vi "Shift  Master_OLD.vi"(8 "error in (no error)":errorcluster) -> (0 "error out":errorcluster)   [LabVIEW 2017]
uses:
  <vilib>/Utility/miscctls.llb/LVRowAndColumnTypeDef.ctl
  <vilib>/Utility/miscctls.llb/LVBoundsTypeDef.ctl
  <vilib>/addons/database/Connection.llb/DB Tools Open Connec (Path).vi
  Globle/Current date.vi
  <vilib>/addons/database/NI_Database_API.lvlib
panel:
  in  "Back 2":bool
  in  "UPDATE":bool
  in  "Shift 3 Stop Time":timestamp format="%<%H-%M-%S>T"
  in  "Shift 2Stop Time":timestamp format="%<%H-%M-%S>T"
  out "Shift 3 Start Time":timestamp format="%<%H-%M-%S>T"
  out "Shift 2 Start Time":timestamp format="%<%H-%M-%S>T"
  in  "Shift 1 Stop Time":timestamp format="%<%H-%M-%S>T"
  in  "Shift 1 Start time":timestamp format="%<%H-%M-%S>T"
  # "Shift Master"
  # "Shift Start Time"
  # "Shift End Time"
  # "Update"
  # "Shift Name"
  # "Shift One"
  # "Shift Two"
  # "Shift Three"
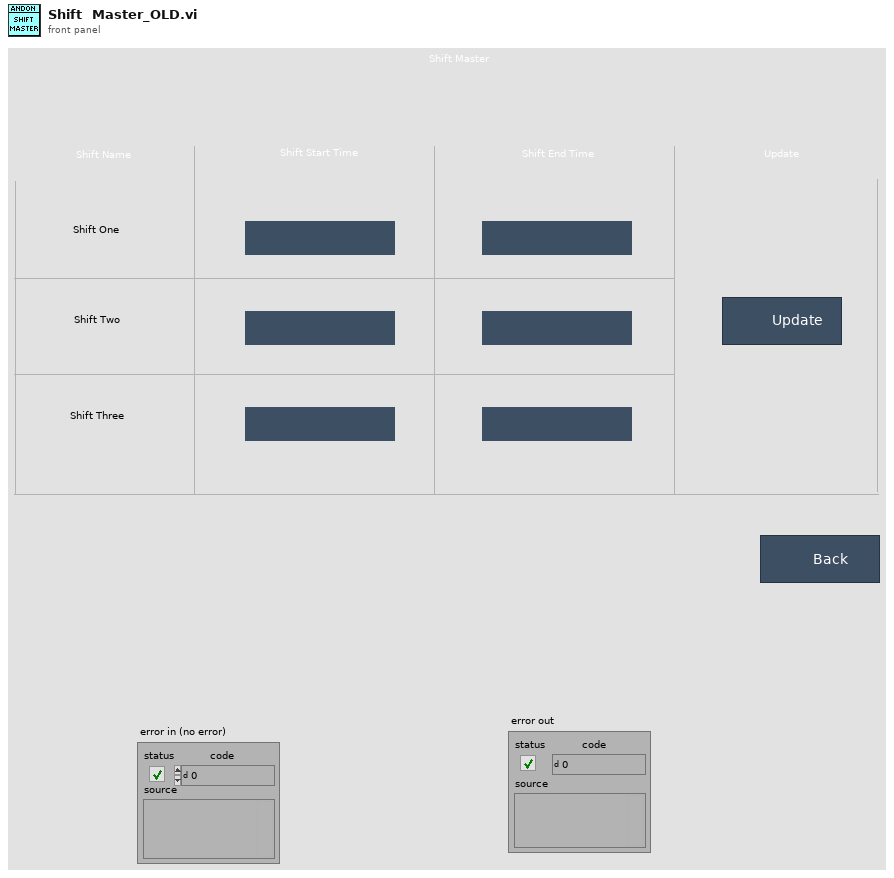
[diagram p1: front panel]
types:
  T1 = typedef "LVBoundsTypeDef.ctl" = cluster{"Width":u32, "Height":u32}
  T2 = typedef "LVRowAndColumnTypeDef.ctl" = cluster{"Row":i32, "Column":i32}
  T3 = typedef "NI_Database_API.lvlib/Conn ObjectReference.ctl" = refnum<k1>
  T4 = cluster{"Shift 3 Start Time":timestamp, "Shift 3 Stop Time ":timestamp}
  T5 = cluster{"Shift 2 Start Time":timestamp, "Shift 2Stop Time":timestamp}
  T6 = cluster{"Shift 1 Start time":timestamp, "Shift 1 Stop Time":timestamp}
  T7 = cluster{"Shift 3 Start Time":timestamp, "Shift 3 Stop Time ":timestamp}[]
  T8 = enum32{"invalid app kind", "Development System", "Run Time System", "Student Edition", "Embedded LabVIEW", "Evaluation", "Custom"}
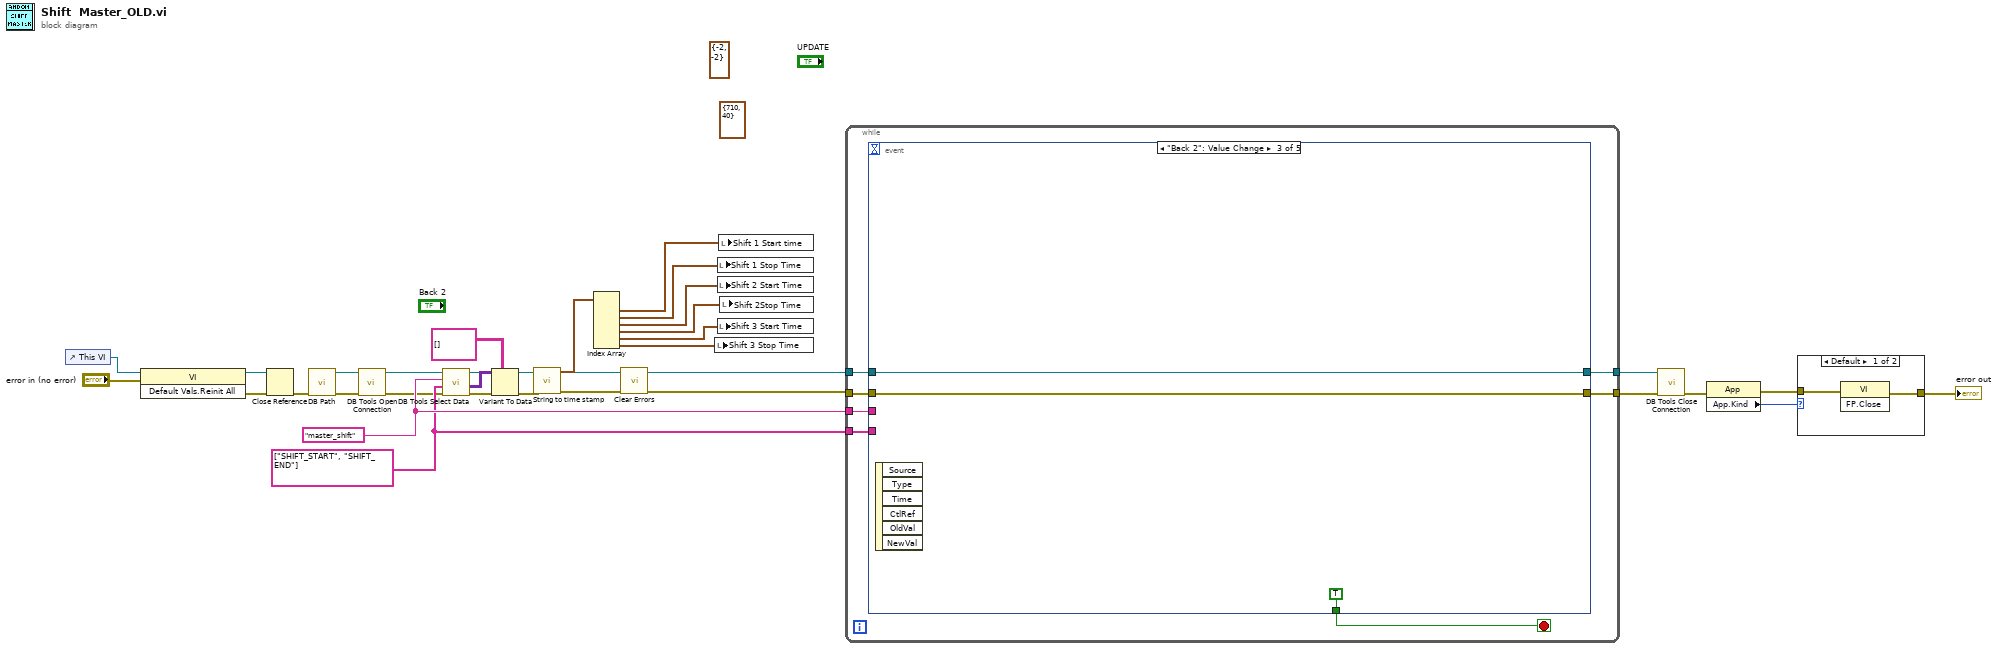
[diagram p0: block diagram]
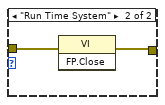
[diagram p2: hidden frame]
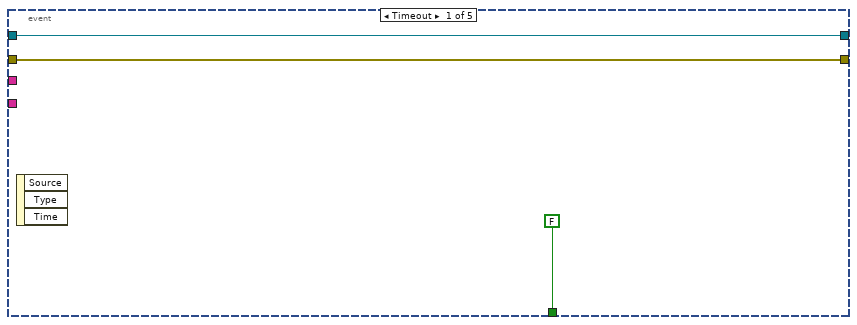
[diagram p3: hidden frame]
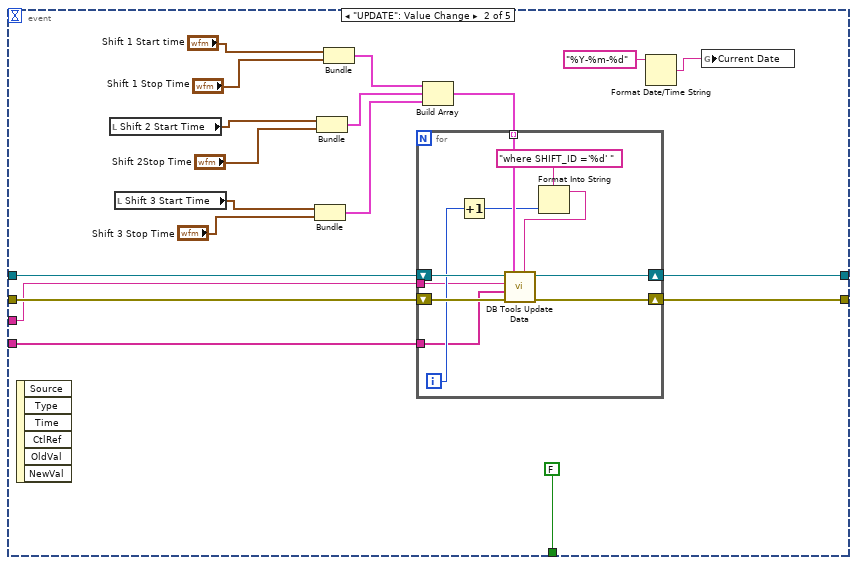
[diagram p4: hidden frame]
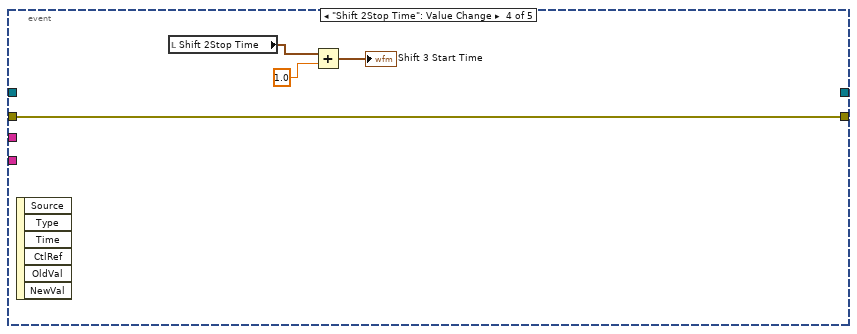
[diagram p5: hidden frame]
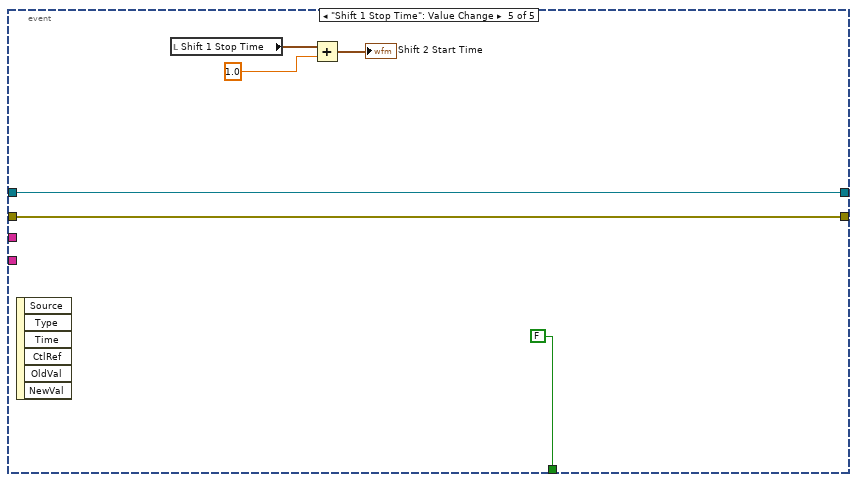
[diagram p6: hidden frame]
diagram:
  w6 = string[] ["SHIFT_START", "SHIFT_END"] ("columns")
  w7 = "master_shift" ("table")
  (unwired) T1 {"Width"=710, "Height"=40} ("Active Cell:Cell Size")
  (unwired) T2 {"Row"=-2, "Column"=-2} ("Active Cell:Active Cell")
  n1 = control-ref of="This VI"() -> (w32:refnum<vi>)
  n2 = invoke class="VI" method="Default Vals.Reinit All"(reference=w32, error in="error in (no error)") -> (reference out=w29:refnum<vi>, error out=w30:errorcluster)  [unwired: 1 in, 1 out]
  n3 = Close Reference(reference=w29, error in (no error)=w30) -> (error out=w25:errorcluster)
  n4 = call "DB Path.vi"("error in"=w25) -> ("error out"=w24:errorcluster, "DB Path"=w23:path)  [unwired: 9 in]
  n5 = call-poly <vilib>:"DB Tools Open Connection.vi"("error in (no error)"=w24, "connection information"=w23) -> ("error out"=w1:errorcluster, "connection reference"=w2:T3)  [unwired: 6 in]
  n6 = call <vilib>:"DB Tools Select Data.vi"("error in (no error)"=w1, "columns"=w6, "table"=w7, "connection reference"=w2) -> ("error out"=w21:errorcluster, "data"=w22:variant[][], "connection reference out"=w11:T3)  [unwired: 2 in]
  n7 = Variant To Data(error in=w21, type=string[][] [], Variant=w22) -> (data=w5:string[][], error out=w19:errorcluster)
  n8 = call "String to time stamp.vi"("error in (no error)"=w19, "Data In"=w5) -> ("error out"=w4:errorcluster, "Time Stamp Out"=w18:timestamp[])  [unwired: 8 in]
  n9 = Index Array(array=w18) -> (element #1=w17:timestamp, element #2=w16:timestamp, element #3=w15:timestamp, element #4=w14:timestamp, element #5=w13:timestamp, element #6=w12:timestamp)  [unwired: 6 in]
  n10 = call <vilib>:"Clear Errors.vi"("error in (no error)"=w4) -> ("error out"=w3:errorcluster)  [unwired: 5 in, 1 out]
  n11 = local write "Shift 3 Stop Time"(w12) -> ()
  n12 = local write "Shift 1 Stop Time"(w16) -> ()
  n13 = local write "Shift 2 Start Time"(w15) -> ()
  n14 = local write "Shift 3 Start Time"(w13) -> ()
  n15 = local write "Shift 1 Start time"(w17) -> ()
  n16 = local write "Shift 2Stop Time"(w14) -> ()
  n17 = while {
    tunnel: w3 -> [w39]
    tunnel: [w37] -> w10
    tunnel: w11 -> [w36]
    tunnel: [w35] -> w8
    tunnel: w7 -> [w34]
    tunnel: w6 -> [w33]
    stop <- w38 stop-if-true
    n18 = event shown="[2] \"Back 2\": Value Change" {
      selector: _ -> [_ _ _ _ _]
      dyn-events: _ -> [_ _ _ _ _]
      timeout: _ -> [_ _ _ _ _]
      tunnel: w39 -> [w41 w52 w74 w79 w83]
      tunnel: [FALSE FALSE TRUE _ FALSE] -> w38
      tunnel: [w41 w46 w74 w79 w83] -> w37
      tunnel: w36 -> [w42 w51 w75 _ w80]
      tunnel: [w42 w45 w75 _ w80] -> w35
      tunnel: w34 -> [_ w50 _ _ _]
      tunnel: w33 -> [_ w49 _ _ _]
      event Timeout {
        n19 = event-data() -> ()  [unwired: 1 in, 3 out]
      }
      event "UPDATE": Value Change {
        n20 = event-data() -> ()  [unwired: 1 in, 6 out]
        n21 = local read "Shift 2 Start Time"() -> (w57:timestamp)
        n22 = local read "Shift 3 Start Time"() -> (w56:timestamp)
        n23 = Bundle("Shift 3 Start Time"=w56, "Shift 3 Stop Time"="Shift 3 Stop Time") -> (w54:T4)  [unwired: 1 in]
        n24 = Bundle("Shift 2 Start Time"=w57, "Shift 2Stop Time"="Shift 2Stop Time") -> (w55:T5)  [unwired: 1 in]
        n25 = Bundle("Shift 1 Start time"="Shift 1 Start time", "Shift 1 Stop Time"="Shift 1 Stop Time") -> (w53:T6)  [unwired: 1 in]
        n26 = Build Array(w53, w55, w54) -> (w48:T7)
        n27 = for {
          tunnel: w50 -> [w62]
          tunnel: w49 -> [w63]
          tunnel: w48 -> [w68] mode=indexing
          shift-right: [w71] -> w46
          shift-left: w52 -> [w72]
          shift-right: [w69] -> w45
          shift-left: w51 -> [w70]
          i -> [w65]
          n28 = Increment(x=w65) -> (x+1=w64:i32)
          n29 = Format Into String(format string="where SHIFT_ID ='%d' ", w64) -> (resulting string=w67:string)  [unwired: 2 in, 1 out]
          n30 = call <vilib>:"DB Tools Update Data.vi"("condition"=w67, "data"=w68, "error in (no error)"=w72, "columns"=w63, "table"=w62, "connection reference"=w70) -> ("error out"=w71:errorcluster, "connection reference out"=w69:T3)  [unwired: 4 in]
        }
        n31 = Format Date/Time String(time format string (%c)="%Y-%m-%d") -> (date/time string=w43:string)  [unwired: 2 in]
        n32 = global write "Current date.vi" "Current Date"(w43) -> ()
      }
      event "Back 2": Value Change {
        n33 = event-data() -> ()  [unwired: 1 in, 6 out]
      }
      event "Shift 2Stop Time": Value Change {
        n34 = event-data() -> ()  [unwired: 1 in, 6 out]
        n35 = local read "Shift 2Stop Time"() -> (w78:timestamp)
        n36 = Add(x=w78, y=1.0) -> (x+y=→"Shift 3 Start Time":timestamp)
      }
      event "Shift 1 Stop Time": Value Change {
        n37 = event-data() -> ()  [unwired: 1 in, 6 out]
        n38 = local read "Shift 1 Stop Time"() -> (w85:timestamp)
        n39 = Add(x=w85, y=1.0) -> (x+y=→"Shift 2 Start Time":timestamp)
      }
    }
  }
  n40 = call <vilib>:"DB Tools Close Connection.vi"("error in (no error)"=w10, "connection reference"=w8) -> ("error out"=w9:errorcluster)  [unwired: 5 in]
  n41 = property class="App"(error in=w9) -> (error out=w27:errorcluster, "App.Kind"=w28:T8)  [unwired: 1 in, 1 out]
  n42 = case shown="Default" w28 {
    tunnel: w27 -> [w87 w89]
    tunnel: [w86 w88] -> w26
    frame Default {
      n43 = invoke class="VI" method="FP.Close"(error in=w87) -> (error out=w86:errorcluster)  [unwired: 2 in, 2 out]
    }
    frame "Run Time System" {
      n44 = invoke class="VI" method="FP.Close"(error in=w89) -> (error out=w88:errorcluster)  [unwired: 2 in, 2 out]
    }
  }
  "error out" <- w26
